vi "Parse Data Out.vi"(0 "Raw Data In":string, 11 "Error In":errorcluster) -> (4 "Data Out":T1 {"CRC" format="%04x"; "Length" format="%02x"; "Command" format="%02x"; "Destination" format="%02x"; "Source" format="%02x"}, 8 "Raw Data Out":string, 15 "Error Out":errorcluster)   [LabVIEW 2023, in "GEA2_Toolkit.lvlib"]
uses:
  library/GEA2_Toolkit.lvlib
  type defs/Data Out.ctl
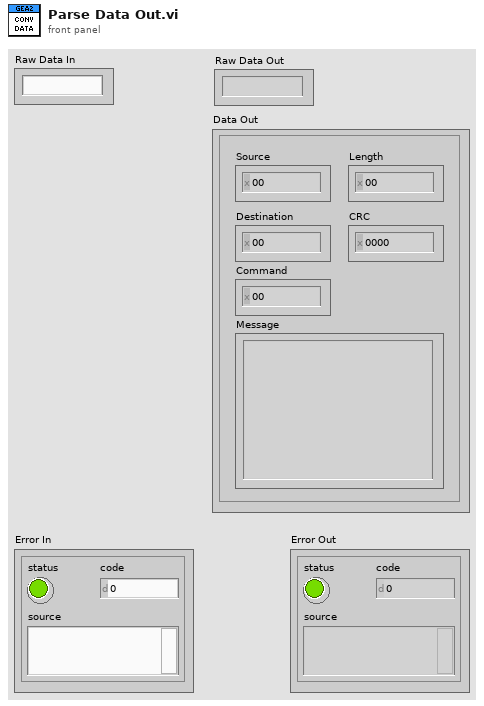
[diagram p1: front panel]
types:
  T1 = typedef "GEA2_Toolkit.lvlib/Data Out.ctl" = cluster{"Source":u8, "Destination":u8, "Command":u8, "Length":u8, "CRC":u16, "Message":string}
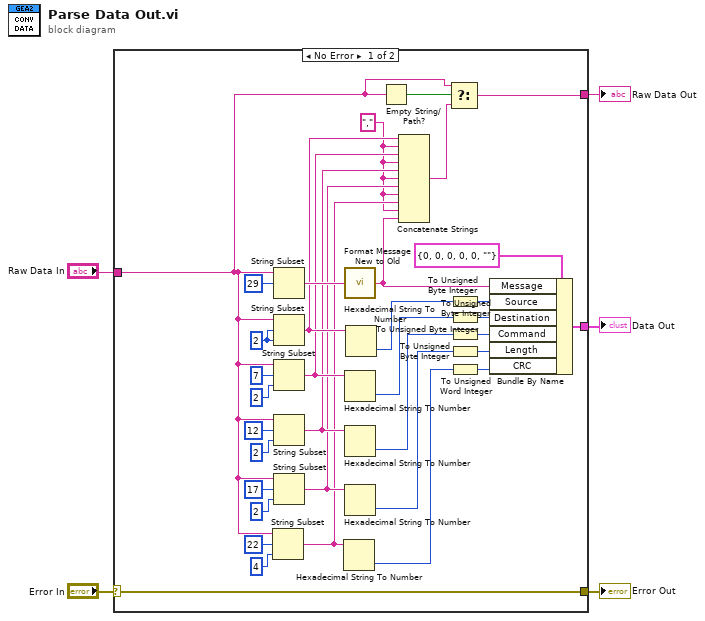
[diagram p0: block diagram]
diagram:
  n1 = case shown="No Error" "Error In" {
    selector: "Error In" -> [w35 w41]
    tunnel: [w35 w41] -> w4
    tunnel: [w27 _] -> w3
    tunnel: "Raw Data In" -> [w8 _]
    tunnel: [w6 _] -> w1
    frame No Error {
      w11 = "," ("string")
      w18 = 2 ("length (rest)")
      n2 = String Subset(string=w8, offset (0)=22, length (rest)=4 ("length (rest)")) -> (substring=w12:string)
      n3 = String Subset(string=w8, offset (0)=29) -> (substring=w17:string)  [unwired: 1 in]
      n4 = String Subset(string=w8, offset (0)=w18, length (rest)=w18) -> (substring=w16:string)
      n5 = String Subset(string=w8, offset (0)=7, length (rest)=2 ("length (rest)")) -> (substring=w15:string)
      n6 = String Subset(string=w8, offset (0)=12, length (rest)=2 ("length (rest)")) -> (substring=w14:string)
      n7 = String Subset(string=w8, offset (0)=17, length (rest)=2 ("length (rest)")) -> (substring=w13:string)
      n8 = Hexadecimal String To Number(string=w12) -> (number=w19:u32)  [unwired: 2 in, 1 out]
      n9 = call "Format Message New to Old.vi"("Raw Message In"=w17) -> ("Conv Message Out"=w10:string)  [unwired: 14 in]
      n10 = Hexadecimal String To Number(string=w15) -> (number=w30:u32)  [unwired: 2 in, 1 out]
      n11 = Hexadecimal String To Number(string=w14) -> (number=w29:u32)  [unwired: 2 in, 1 out]
      n12 = Hexadecimal String To Number(string=w13) -> (number=w23:u32)  [unwired: 2 in, 1 out]
      n13 = Hexadecimal String To Number(string=w16) -> (number=w34:u32)  [unwired: 2 in, 1 out]
      n14 = Empty String/Path?(string/path=w8) -> (empty?=w9:bool)
      n15 = Concatenate Strings(w16, w11, w15, w11, w14, w11, w13, w11, w12, w11, w10) -> (w7:string)
      n16 = Select(t=w8, s=w9, f=w7) -> (s? t:f=w6:string)
      n17 = To Unsigned Byte Integer(number=w34) -> (unsigned 8bit integer=w33:u8)
      n18 = To Unsigned Byte Integer(number=w30) -> (unsigned 8bit integer=w32:u8)
      n19 = To Unsigned Byte Integer(number=w29) -> (unsigned 8bit integer=w31:u8)
      n20 = To Unsigned Byte Integer(number=w23) -> (unsigned 8bit integer=w24:u8)
      n21 = To Unsigned Word Integer(number=w19) -> (unsigned 16bit integer=w22:u16)
      n22 = Bundle By Name(cluster=T1 {"Source"=0, "Destination"=0, "Command"=0, "Length"=0, "CRC"=0, "Message"=""} ("Data Out"), "Message"=w10, "Source"=w33, "Destination"=w32, "Command"=w31, "Length"=w24, "CRC"=w22) -> (w27:T1)
    }
    frame Error {
    }
  }
  "Error Out" <- w4
  "Data Out" <- w3
  "Raw Data Out" <- w1
